vi "GoBang_CheckArray.vi"(0 "5x5 array":u8[][](array[numeric])) -> (1 "white won":bool, 2 "black won":bool, 3 "game over":bool)   [LabVIEW 2013, in "GoBang.lvlib"]
uses:
  GoBang.lvlib
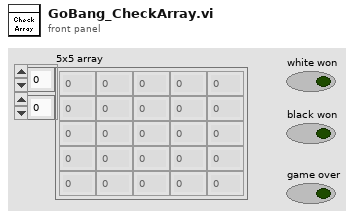
[diagram p1: front panel]
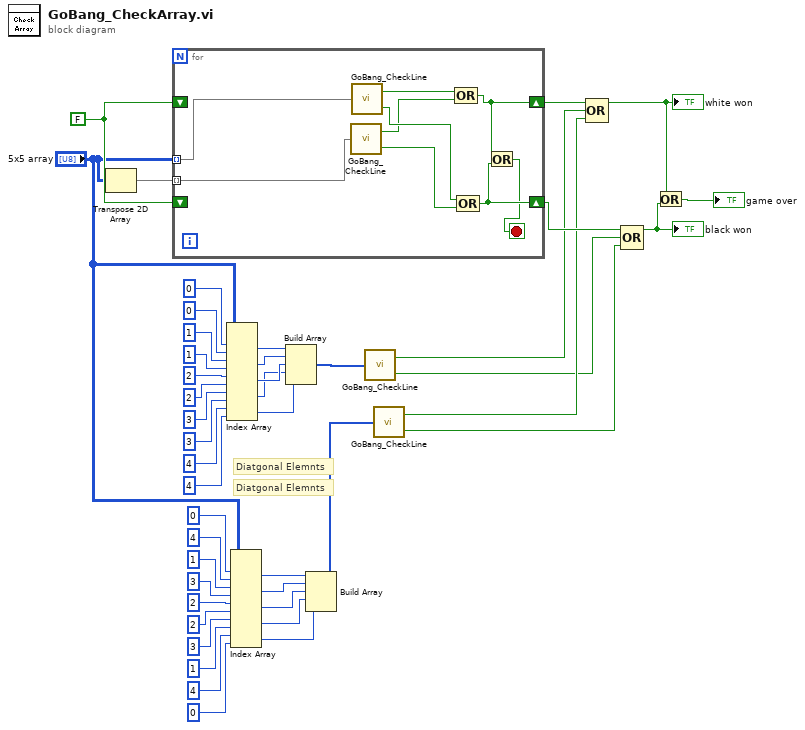
[diagram p0: block diagram]
diagram:
  w44 = FALSE
  # "Diatgonal Elemnts"
  # "Diatgonal Elemnts"
  n1 = Transpose 2D Array(2D array="5x5 array") -> (transposed array=w40:u8[][])
  n2 = for {
    tunnel: "5x5 array" -> [w49] mode=indexing
    shift-right: [w47] -> w43
    shift-left: w44 -> [_]
    shift-right: [w46] -> w42
    shift-left: w44 -> [_]
    tunnel: w40 -> [w48] mode=indexing
    stop <- w45 stop-if-true
    n3 = call "GoBang_CheckLine.vi"("line with 5 elements"=w48) -> ("White won"=w51:bool, "Black won"=w50:bool)
    n4 = call "GoBang_CheckLine.vi"("line with 5 elements"=w49) -> ("White won"=w52:bool, "Black won"=w53:bool)
    n5 = Compound Arithmetic op=OR(w52, w51) -> (w47:bool)
    n6 = Compound Arithmetic op=OR(w53, w50) -> (w46:bool)
    n7 = Or(x=w47, y=w46) -> (x .or. y?=w45:bool)
  }
  n8 = Index Array(array="5x5 array", index (row) #1=0 ("index (row)"), index (col) #1=0 ("disabled index (col)"), index (row) #2=1 ("index (row)"), index (col) #2=1 ("disabled index (col)"), index (row) #3=2 ("index (row)"), index (col) #3=2 ("disabled index (col)"), index (row) #4=3 ("index (row)"), index (col) #4=3 ("disabled index (col)"), index (row) #5=4 ("index (row)"), index (col) #5=4 ("disabled index (col)")) -> (element #1=w29:u8, element #2=w28:u8, element #3=w27:u8, element #4=w26:u8, element #5=w25:u8)
  n9 = Index Array(array="5x5 array", index (row) #1=0 ("index (row)"), index (col) #1=4 ("disabled index (col)"), index (row) #2=1 ("index (row)"), index (col) #2=3 ("disabled index (col)"), index (row) #3=2 ("index (row)"), index (col) #3=2 ("disabled index (col)"), index (row) #4=3 ("index (row)"), index (col) #4=1 ("disabled index (col)"), index (row) #5=4 ("index (row)"), index (col) #5=0 ("disabled index (col)")) -> (element #1=w12:u8, element #2=w10:u8, element #3=w9:u8, element #4=w8:u8, element #5=w7:u8)
  n10 = Build Array(w29, w28, w27, w26, w25) -> (w24:u8[])
  n11 = Build Array(w12, w10, w9, w8, w7) -> (w11:u8[])
  n12 = call "GoBang_CheckLine.vi"("line with 5 elements"=w24) -> ("White won"=w5:bool, "Black won"=w3:bool)
  n13 = call "GoBang_CheckLine.vi"("line with 5 elements"=w11) -> ("White won"=w4:bool, "Black won"=w2:bool)
  n14 = Compound Arithmetic op=OR(w43, w5, w4) -> (w6:bool)
  "white won" <- w6
  n15 = Compound Arithmetic op=OR(w42, w3, w2) -> (w1:bool)
  "black won" <- w1
  n16 = Or(x=w6, y=w1) -> (x .or. y?=→"game over":bool)
